vi "Write Text.vi"(8 "error in (no error)":errorcluster, 9 "timeout ms (5000)":i32=5000, 10 "String":string, 11 "WebSocket in":refnum<class "WebSocket.lvclass">) -> (0 "error out":errorcluster, 3 "WebSocket out":refnum<class "WebSocket.lvclass">)   [LabVIEW 2013, in "WebSockets.lvlib" / "WebSocket.lvclass"]
uses:
  WebSocket.lvclass
  Opcodes.ctl
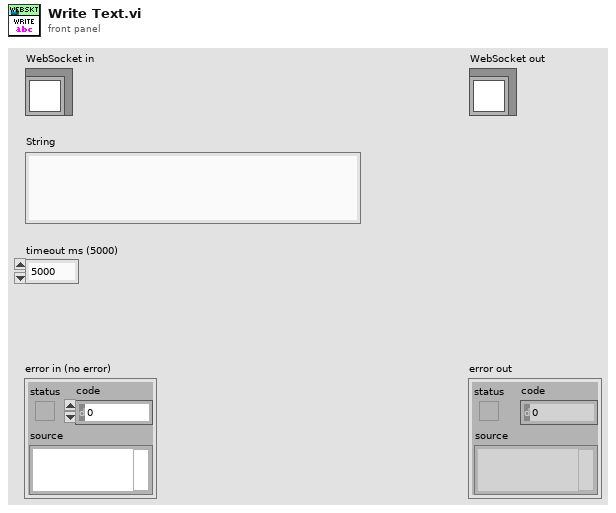
[diagram p1: front panel]
types:
  T1 = typedef "WebSockets.lvlib/WebSocket.lvclass/Opcodes.ctl" = u8
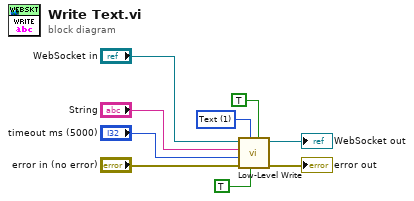
[diagram p0: block diagram]
diagram:
  w1 = T1 1 items=["Cont. Frame"=0, "Text"=1, "Binary"=2, "Close Frame"=8, "Ping"=9, "Pong"=10] ("Opcode (Text)")
  n1 = call "Low-Level Write.vi"("Finished? (True)"=TRUE, "Mask payload?"=TRUE, "Opcode (Text)"=w1, "error in (no error)"="error in (no error)", "timeout ms (5000)"="timeout ms (5000)", "Data"="String", "WebSockets in"="WebSocket in") -> ("error out"=→"error out":errorcluster, "WebSockets out"=→"WebSocket out":refnum<class "WebSocket.lvclass">)  [unwired: 3 in]
